vi "GetBitfilePath.vi"(11 "productName":string) -> (3 "bitfile path":path)   [LabVIEW 2017, in "cRIODetectHW.lvlib"]
uses:
  <vilib>/addons/cRIODetectHW/cRIODetectHW.lvlib
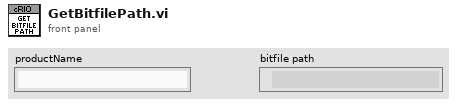
[diagram p1: front panel]
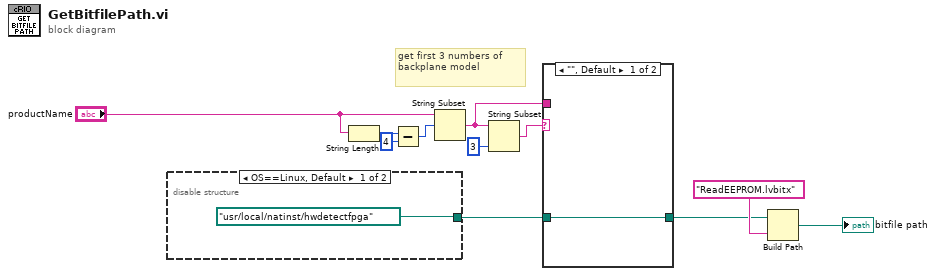
[diagram p0: block diagram]
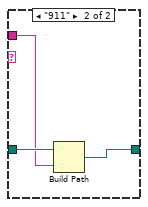
[diagram p2: hidden frame]
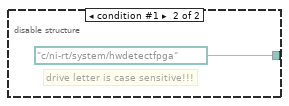
[diagram p3: hidden frame]
diagram:
  # "get first 3 numbers of backplane model"
  n1 = disable-structure shown="OS==Linux, Default" {
    disable-tunnel: [path "/usr/local/natinst/hwdetectfpga" path "c:/ni-rt/system/hwdetectfpga"] -> w8
    frame condition #0 (active) {
    }
    frame condition #1 {
      # "drive letter is case sensitive!!!"
    }
  }
  n2 = String Length(string="productName") -> (length=w1:i32)
  n3 = Subtract(x=w1, y=4) -> (x-y=w3:i32)
  n4 = String Subset(string="productName", offset (0)=w3) -> (substring=w5:string)  [unwired: 1 in]
  n5 = String Subset(string=w5, length (rest)=3 ("length (rest)")) -> (substring=w6:string)  [unwired: 1 in]
  n6 = case shown="\"\", Default" w6 {
    tunnel: w5 -> [_ w15]
    tunnel: w8 -> [w14 w17]
    tunnel: [w14 w16] -> w9
    frame "", Default {
    }
    frame "911" {
      n7 = Build Path(base path=w17, name or relative path=w15) -> (appended path=w16:path)
    }
  }
  n8 = Build Path(base path=w9, name or relative path="ReadEEPROM.lvbitx") -> (appended path=→"bitfile path":path)
